vi "ExpandList.vi"(11 "Tags in":string[](array[string])) -> (1 "Tags":string[](array[string]), 3 "List Paths":path[](array[path]))   [LabVIEW 2022 SP3]
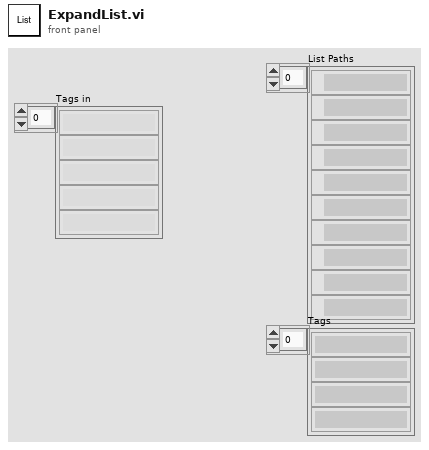
[diagram p1: front panel]
types:
  T1 = typedef "Curtin1_Label.ctl" = cluster{"Show?":bool, "Name":string, "Color":u32, "Path":path, "Show Notes":bool}
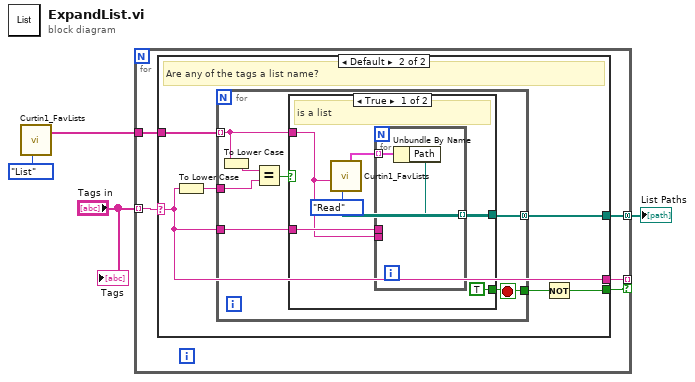
[diagram p0: block diagram]
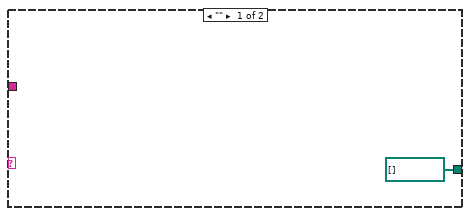
[diagram p2: hidden frame]
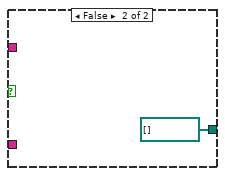
[diagram p3: hidden frame]
diagram:
  n1 = call "Curtin1_FavLists.vi"("Task"=enum16{"Save", "Read", "List", "Delete"}."List") -> ("Lists"=w3:string[])  [unwired: 7 in, 3 out]
  n2 = for {
    tunnel: "Tags in" -> [w7] mode=indexing
    tunnel: [w9] -> w2 mode=concatenating
    tunnel: w3 -> [w8]
    tunnel: [w6] -> _ mode=indexing if=w5
    n3 = case shown="Default" w7 {
      selector: w7 -> [_ w11]
      tunnel: [path[] [] w14] -> w9
      tunnel: w8 -> [_ w15]
      tunnel: [_ w11] -> w6
      tunnel: [_ w12] -> w5
      frame "" {
      }
      frame Default {
        # "Are any of the tags a list name?"
        n4 = To Lower Case(string=w11) -> (all lower case string=w16:string)
        n5 = for {
          tunnel: w16 -> [w18]
          tunnel: [w23] -> w14 mode=concatenating
          tunnel: w15 -> [w20] mode=indexing
          tunnel: [w22] -> w13
          tunnel: w11 -> [w21]
          stop <- w22 stop-if-true
          n6 = To Lower Case(string=w20) -> (all lower case string=w19:string)
          n7 = Equal?(x=w19, y=w18) -> (x = y?=w17:bool)
          n8 = case shown="True" w17 {
            tunnel: [w29 path[] []] -> w23
            tunnel: w20 -> [w25 _]
            tunnel: [TRUE _] -> w22
            tunnel: w21 -> [w27 _]
            frame True {
              # "is a list"
              n9 = call "Curtin1_FavLists.vi"("Task"=enum16{"Save", "Read", "List", "Delete"}."Read", "List Name"=w25) -> ("Files Out"=w24:T1[])  [unwired: 6 in, 3 out]
              n10 = for {
                tunnel: [w30] -> w29 mode=indexing
                tunnel: w25 -> [_]
                tunnel: w27 -> [_]
                tunnel: w24 -> [w31] mode=indexing
                n11 = Unbundle By Name(w31) -> ("Path"=w30:path)
              }
            }
            frame False {
            }
          }
        }
        n12 = Not(x=w13) -> (.not. x?=w12:bool)
      }
    }
  }
  "List Paths" <- w2
  "Tags" <- "Tags in"
